vi "Get Current LV Dir.vi"(8 "Error In":errorcluster) -> (0 "Error Out":errorcluster, 3 "This LV Directory":path)   [LabVIEW 2011, in "LMH-Toolbox.lvlib" / "LMH-Common.lvlib"]
doc: "Get the absolute path of LabVIEW directory for the version of LabVIEW this VI is executed in."
uses:
  LMH-Common.lvlib
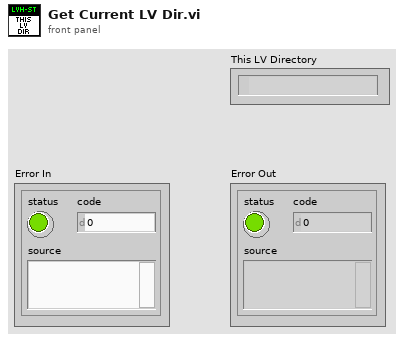
[diagram p1: front panel]
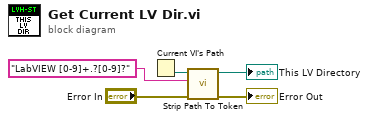
[diagram p0: block diagram]
diagram:
  n1 = Current VI's Path() -> (path=w4:path)
  n2 = call "Strip Path To Token.vi"("Error In"="Error In", "Token (Regex)"="LabVIEW [0-9]+.?[0-9]?", "Path"=w4) -> ("Error Out"=→"Error Out":errorcluster, "Stripped Path"=→"This LV Directory":path)  [unwired: 6 in, 1 out]
